vi "Columns.vi"() -> (2 "Columns":T1)   [LabVIEW 2020, in "tests.lvlib" / "LiveDemo.lvclass"]
uses:
  LiveDemo.lvclass
  Columns.ctl
  <vilib>/IlluminatedG/IG Conditum Base/Conditum/Columns/Integer/Integer.lvclass
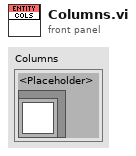
[diagram p1: front panel]
types:
  T1 = typedef "tests.lvlib/LiveDemo.lvclass/Columns.ctl" = cluster{"<Placeholder>":refnum<class "Integer.lvclass">}
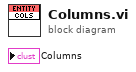
[diagram p0: block diagram]
diagram:
